vi "START2.vi"() -> ()   [LabVIEW 2024]
uses:
  <vilib>/Utility/file.llb/Read Delimited Spreadsheet (DBL).vi
panel:
  out "Rotations Per Minute Waveform":dbl[](graph)
  out "Flow Rate Waveform":dbl[](graph)
  in  "stop":bool
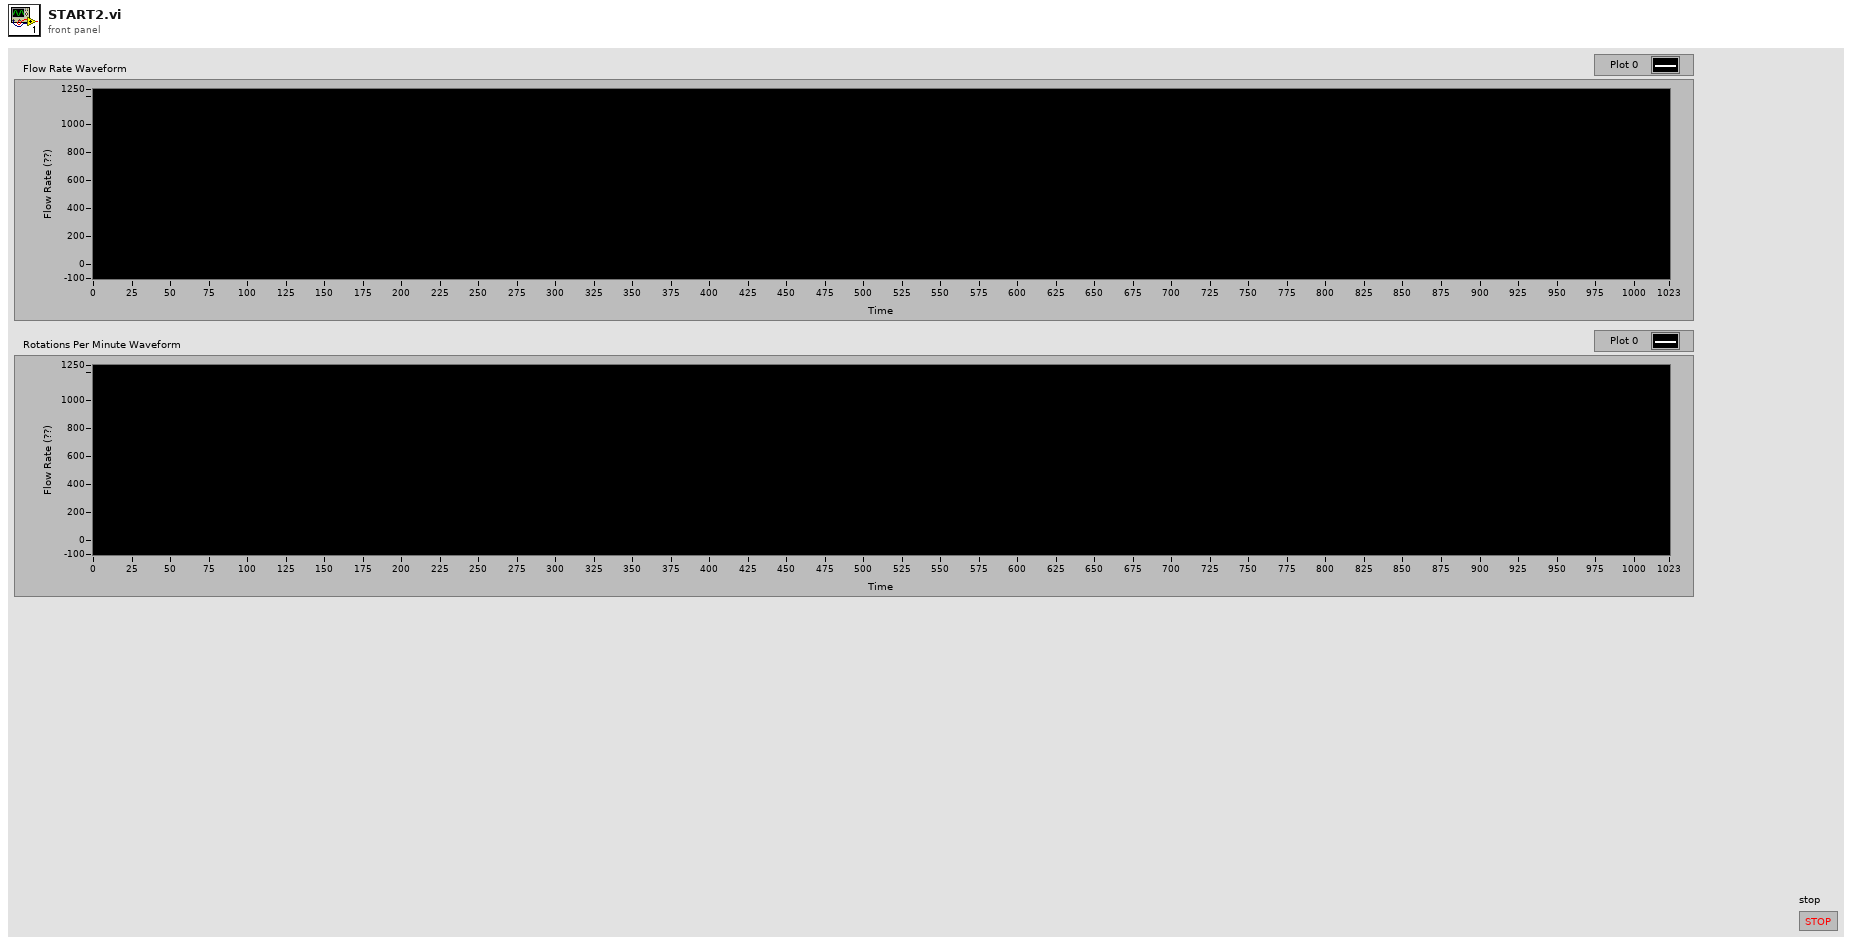
[diagram p1: front panel]
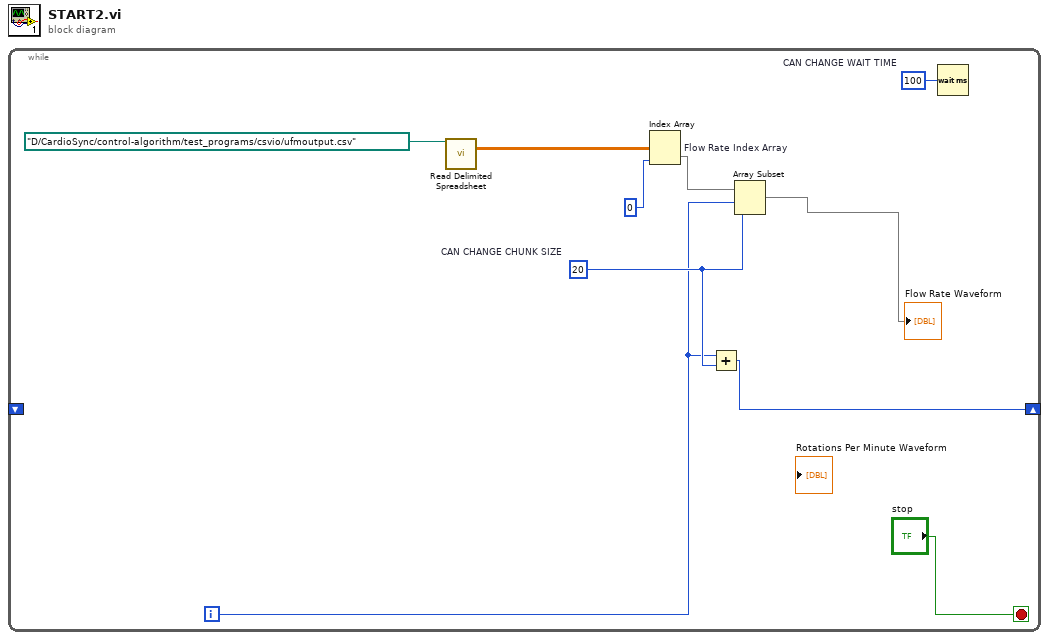
[diagram p0: block diagram]
diagram:
  n1 = while {
    shift-right: [w3] -> _
    shift-left: _ -> [_]
    i -> [w2]
    stop <- "stop" stop-if-true
    w5 = u32 100  # CAN CHANGE WAIT TIME
    w6 = 20  # CAN CHANGE CHUNK SIZE
    n2 = call-poly <vilib>:"Read Delimited Spreadsheet.vi"("file path (dialog if empty)"=path "D:/CardioSync/control-algorithm/test_programs/csvio/ufmoutput.csv") -> ("all rows"=w8:dbl[][])  [unwired: 9 in, 5 out]
    n3 = Index Array "Flow Rate Index Array"(array=w8, index (col)=0 ("disabled index (col)")) -> (element=w7:dbl[])  [unwired: 1 in]
    n4 = Add(x=w2, y=w6) -> (x+y=w3:i32)
    n5 = Array Subset(array=w7, index=w2, length=w6) -> (→"Flow Rate Waveform":dbl[])
    n6 = Wait (ms)(milliseconds to wait=w5) -> ()  [unwired: 1 out]
  }
